vi "Get Ordered DO Channels_Status_IO.vi"(8 "error in (no error)":errorcluster, 11 "IO in":refnum<class "IO.lvclass">) -> (0 "error out":errorcluster, 2 "Ordered DO Channels":T1[](array[typedef]), 3 "IO out":refnum<class "IO.lvclass">)   [LabVIEW 2022 SP3, in "IO.lvclass"]
uses:
  IO.lvclass
  Typedefs/ICP2-DO Channel Names.ctl
  IO.lvclass/IO.ctl
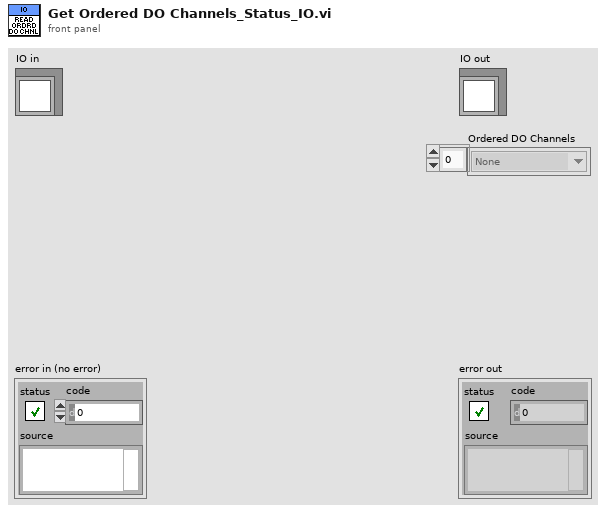
[diagram p1: front panel]
types:
  T1 = typedef "IO.lvclass/ICP2-DO Channel Names.ctl" = enum16{"None", "Meniscus Valve Open - R1", "Meniscus Valve Open - R2", "Meniscus Valve Open - R3", "Meniscus Valve Open - R4", "Meniscus Valve Open - R5", "Meniscus Valve Open - R6", "Ink Flow Valve Open - R1", "Ink Flow Valve Open - R2", "Ink Flow Valve Open - R3", "Ink Flow Valve Open - R4", "Ink Flow Valve Open - R5", "Ink Flow Valve Open - R6", "SW_LED - Ink Valve - R1", "SW_LED - Ink Valve - R2", "SW_LED - Ink Valve - R3", "Recirc Pump On - R1", "Recirc Pump On - R2", "Recirc Pump On - R3", "Recirc Pump On - R4", "Recirc Pump On - R5", "Recirc Pump On - R6", "SW_LED - Ink Valve - R4", "SW_LED - Ink Valve - R5", "SW_LED - Ink Valve - R6"}
  T2 = typedef "IO.lvclass/Private Data.ctl" = cluster{"UserEvents":T3, "All Dependencies":cluster{"Class References":refnum<class>[], "Class Names":string[]}, "Status":T4}
  T3 = typedef "IO.lvclass/UserEvents.ctl" = cluster{"API Incoming Event":refnum<user-event>, "API Executed Event":refnum<user-event>, "API Return Event":refnum<user-event>, "Status Changed Event":refnum<user-event>}
  T4 = typedef "IO.lvclass/Status Cluster.ctl" = cluster{"Device Data":variant, "Ordered ICP2-DI Channels":T5[], "Ordered ICP2-DO Channels":T6[]}
  T5 = typedef "IO.lvclass/DI Channel Names.ctl" = enum16{"None", "SW - Ink Valve - R1", "SW - Ink Valve - R2", "SW - Ink Valve - R3", "SW - Ink Valve - R4", "SW - Ink Valve - R5", "SW - Ink Valve - R6", "SW - COVER INPUT SIDE", "SW - COVER OUTPUT SIDE", "SW - Purge - R1", "SW - Purge - R2", "SW - Purge - R3", "SW - Purge - R4", "SW - Purge - R5", "SW - Purge - R6"}
  T6 = typedef "IO.lvclass/DO Channel Names.ctl" = enum16{"None", "Meniscus Valve Open - R1", "Meniscus Valve Open - R2", "Meniscus Valve Open - R3", "Meniscus Valve Open - R4", "Meniscus Valve Open - R5", "Meniscus Valve Open - R6", "Ink Flow Valve Open - R1", "Ink Flow Valve Open - R2", "Ink Flow Valve Open - R3", "Ink Flow Valve Open - R4", "Ink Flow Valve Open - R5", "Ink Flow Valve Open - R6", "SW_LED - Ink Valve - R1", "SW_LED - Ink Valve - R2", "SW_LED - Ink Valve - R3", "Recirc Pump On - R1", "Recirc Pump On - R2", "Recirc Pump On - R3", "Recirc Pump On - R4", "Recirc Pump On - R5", "Recirc Pump On - R6", "SW_LED - Ink Valve - R4", "SW_LED - Ink Valve - R5", "SW_LED - Ink Valve - R6"}
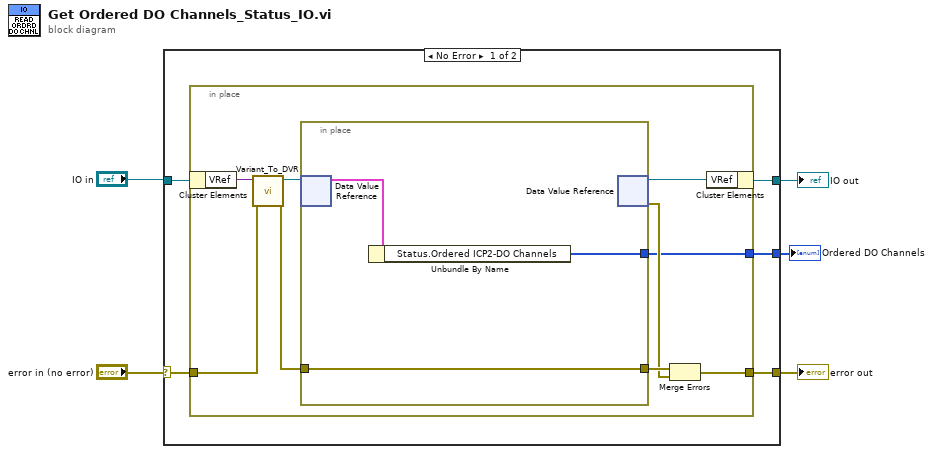
[diagram p0: block diagram]
diagram:
  n1 = case shown="No Error" "error in (no error)" {
    selector: "error in (no error)" -> [w7 w24]
    tunnel: [w9 w24] -> w3
    tunnel: [w10 w23] -> w2
    tunnel: "IO in" -> [w8 w23]
    tunnel: [w6 _] -> w1
    frame No Error {
      n2 = in-place {
        in-place-border: w7 -> [w17]
        in-place-border: [w13] -> w9
        in-place-border: [w11] -> w6
        n3 = in-place-cluster #1(w8) -> ("VRef"=w19:variant)
        n4 = call "Variant_To_DVR.vi"("error in (no error)"=w17, "Variant"=w19) -> ("error out"=w16:errorcluster, "DVR"=w18:refnum<data-value>)  [unwired: 8 in]
        n5 = in-place {
          in-place-border: w16 -> [w21]
          in-place-border: [w21] -> w15
          in-place-border: [w20] -> w11
          n6 = in-place-dvr #2(w18) -> (w22:T2)  [unwired: 1 out]
          n7 = Unbundle By Name(w22) -> ("Status.Ordered ICP2-DO Channels"=w20:T6[])
          n8 = in-place-dvr #2() -> (w12:refnum<data-value>, w14:errorcluster)  [unwired: 1 in]
        }
        n9 = Merge Errors(w15, w14) -> (w13:errorcluster)
        n10 = in-place-cluster #1("VRef"=w12) -> (w10:refnum<class "IO.lvclass">)
      }
    }
    frame Error {
    }
  }
  "error out" <- w3
  "IO out" <- w2
  "Ordered DO Channels" <- w1
